vi "Accumulated Correlation 2D.vi"(4 "Microphone Coordinates (cm, rad)":cluster{"r":dbl, "theta":dbl}[](array[cluster]), 5 "Ny":i32=16, 6 "Radius (cm)":dbl=123.4 format="%#_13g", 7 "Nx":i32=16, 8 "Sound Velocity (cm/s)":dbl=576000.0, 9 "Sampling Rate":i32=500000, 11 "Waveforms":waveform(dbl)[](array[waveform])) -> (2 "Source Coordinates (cm, cm)":cluster{"x":dbl, "y":dbl})   [LabVIEW 2013]
uses:
  <vilib>/Waveform/WDTOps.llb/WDT Index Channel DBL.vi
  <vilib>/Analysis/2dsp.llb/1D Cross Correlation (DBL).vi
  <vilib>/Analysis/NI_AALPro.lvlib
panel:
  out "Rxy 2":dbl[][][](array[numeric])
  out "subarray 2":dbl[](array[numeric])
  out "size(s) 2":i32
  out "Rxy":dbl[](array[numeric])
  out "y Coordinates":dbl[](array[numeric])
  out "x Coordinates":dbl[](array[numeric])
  out "Cross Corr.\n1/2 Length":i32
  out "dy":dbl
  out "dx":dbl
  out "Signals":waveform(dbl)[](graph)
  out "subarray":dbl[][](array[numeric])
  out "size(s)":i32[](array[numeric])
  out "Correlation":dbl[][](graph)
  out "Lag Matrix":dbl[][](array[numeric])
  # "Inputs and Outputs"
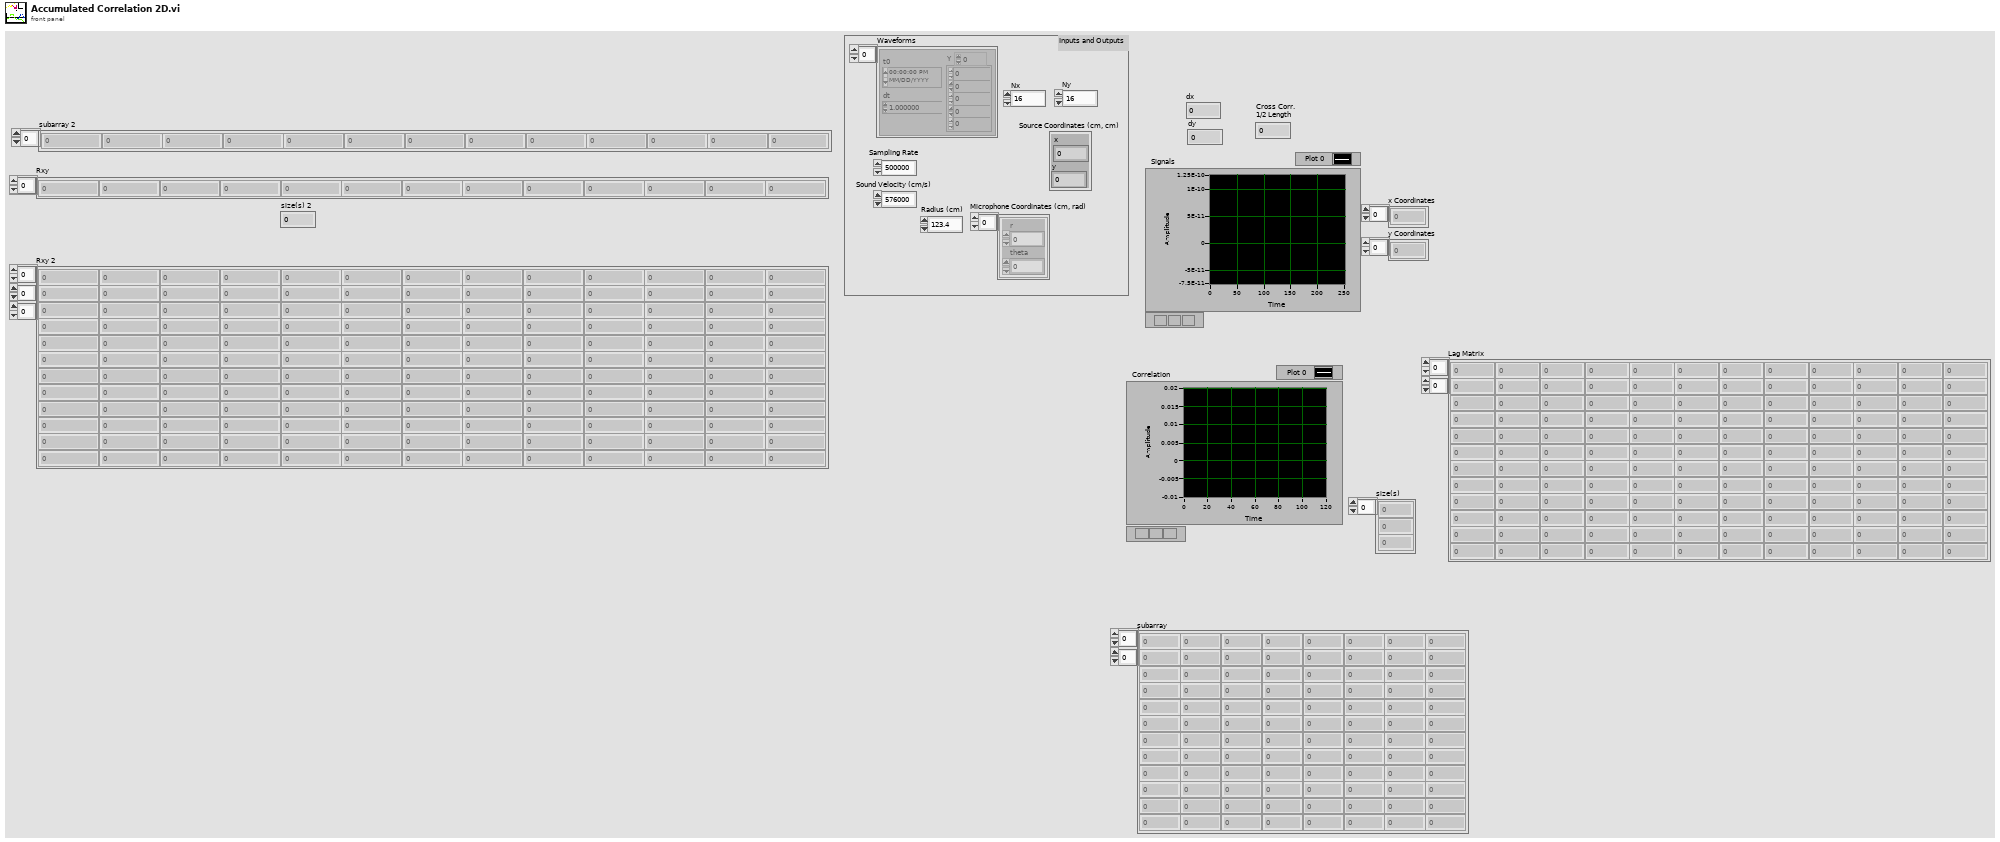
[diagram p1: front panel]
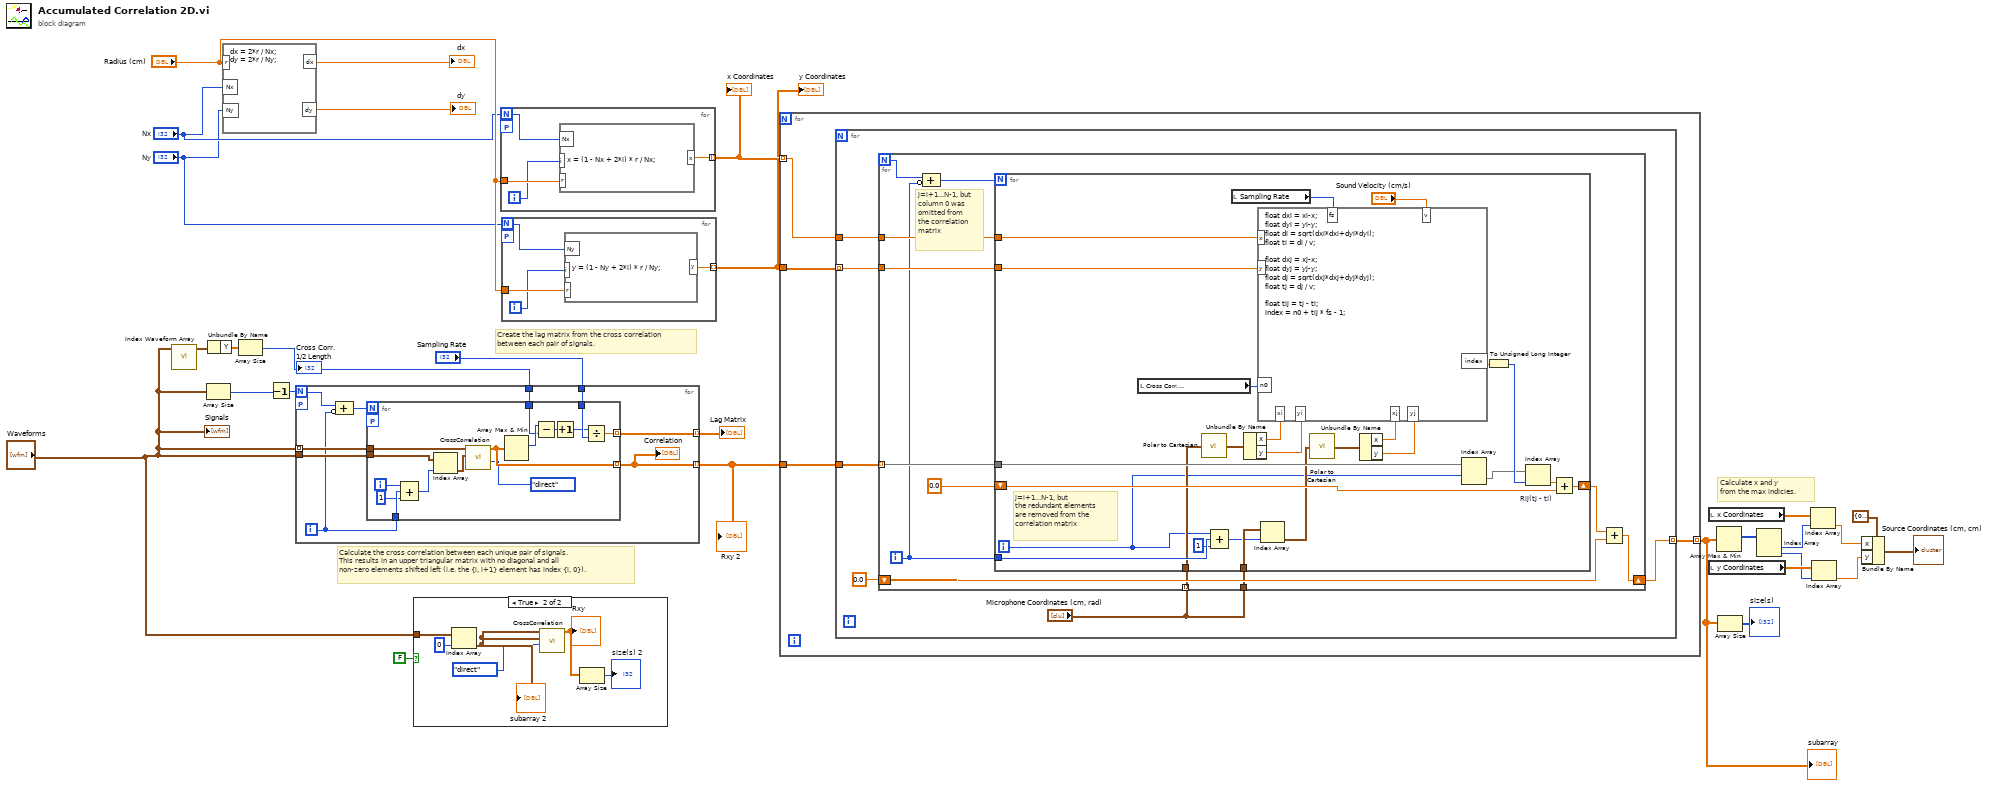
[diagram p0: block diagram]
diagram:
  # "Calculate the cross correlation between each unique pair of signals.\nThis results in an upper triangular matrix with no diagonal and all\nnon-zero elements shifted left (i.e. the {i, i+1} element has index {i, 0})."
  # "Create the lag matrix from the cross correlation\nbetween each pair of signals."
  # "Calculate x and y\nfrom the max indicies."
  n1 = call-poly <vilib>:"Index Waveform Array.vi"("waveform array"="Waveforms") -> ("waveform"=w3:waveform(dbl))  [unwired: 9 in, 1 out]
  n2 = Array Size ("Size(s)")(array="Waveforms") -> (size(s)=w5:i32)
  n3 = Unbundle By Name(w3) -> ("Y"=w2:dbl[])
  n4 = formula code="dx = 2*r / Nx;\ndy = 2*r / Ny;"("r"="Radius (cm)", "Nx"="Nx", "Ny"="Ny") -> ("dx"=→"dx":dbl, "dy"=→"dy":dbl)
  n5 = Array Size(array=w2) -> (size(s)=w1:i32)
  "Cross Corr.\n1/2 Length" <- w1
  n6 = Decrement(x=w5) -> (x-1=w9:i32)
  n7 = for {
    N: w9 -> [w30]
    tunnel: "Waveforms" -> [w33] mode=indexing
    tunnel: "Waveforms" -> [w37]
    tunnel: "Sampling Rate" -> [w36]
    tunnel: [w35] -> w28 mode=indexing
    tunnel: [w34] -> w10 mode=indexing
    tunnel: w1 -> [w32]
    workers-P: _ -> [_]
    i -> [w29]
    n8 = Compound Arithmetic op=ADD(w30, invert w29) -> (w31:i32)
    n9 = for {
      N: w31 -> [_]
      tunnel: w37 -> [w40]
      tunnel: w33 -> [w52]
      tunnel: w36 -> [w51]
      tunnel: [w50] -> w35 mode=indexing
      tunnel: [w47] -> w34 mode=indexing
      tunnel: w32 -> [w45]
      tunnel: w29 -> [w42]
      workers-P: _ -> [_]
      i -> [w43]
      n10 = Compound Arithmetic op=ADD(w43, w42, 1 ("value")) -> (w41:i32)
      n11 = Index Array(array=w40, index=w41) -> (element=w39:waveform(dbl))
      n12 = call-poly <vilib>:"CrossCorrelation.vi"("algorithm"=enum32{"direct", "frequency domain"}."direct", "Y"=w39, "X"=w52) -> ("Rxy"=w47:dbl[])  [unwired: 7 in, 1 out]
      n13 = Array Max & Min(array=w47) -> (max index (indices)=w46:i32)  [unwired: 3 out]
      n14 = Subtract(x=w46, y=w45) -> (x-y=w49:i32)
      n15 = Increment(x=w49) -> (x+1=w48:i32)
      n16 = Divide(x=w48, y=w51) -> (x/y=w50:dbl)
    }
    "Correlation" <- w34
  }
  "Lag Matrix" <- w28
  "Rxy 2" <- w10
  n17 = case shown="True" FALSE {
    tunnel: "Waveforms" -> [_ w58]
    frame False {
    }
    frame True {
      n18 = Index Array(array=w58, index=0 ("index (row)")) -> (element=w56:waveform(dbl))
      "subarray 2" <- w56
      n19 = call-poly <vilib>:"CrossCorrelation.vi"("algorithm"=enum32{"direct", "frequency domain"}."direct", "Y"=w56, "X"=w56) -> ("Rxy"=w54:dbl[])  [unwired: 7 in, 1 out]
      "Rxy" <- w54
      n20 = Array Size(array=w54) -> (size(s)=→"size(s) 2":i32)
    }
  }
  n21 = for {
    N: "Nx" -> [w59]
    tunnel: "Radius (cm)" -> [w62]
    tunnel: [w60] -> w18 mode=indexing
    workers-P: _ -> [_]
    i -> [w61]
    n22 = formula code="x = (1 - Nx + 2*i) * r / Nx;"("r"=w62, "i"=w61, "Nx"=w59) -> ("x"=w60:dbl)
  }
  "x Coordinates" <- w18
  n23 = for {
    N: "Ny" -> [w63]
    tunnel: "Radius (cm)" -> [w66]
    tunnel: [w64] -> w17 mode=indexing
    workers-P: _ -> [_]
    i -> [w65]
    n24 = formula code="y = (1 - Ny + 2*i) * r / Ny;"("r"=w66, "i"=w65, "Ny"=w63) -> ("y"=w64:dbl)
  }
  "y Coordinates" <- w17
  n25 = for {
    tunnel: [w70] -> w25 mode=indexing
    tunnel: w10 -> [w69]
    tunnel: w18 -> [w67] mode=indexing
    tunnel: w17 -> [w68]
    n26 = for {
      tunnel: [w75] -> w70 mode=indexing
      tunnel: w69 -> [w74]
      tunnel: w68 -> [w72] mode=indexing
      tunnel: w67 -> [w71]
      n27 = for {
        N -> [w81]
        shift-right: [w86] -> w75
        shift-left: 0.0 -> [w87]
        tunnel: "Microphone Coordinates (cm, rad)" -> [w85] mode=indexing
        tunnel: "Microphone Coordinates (cm, rad)" -> [w80]
        tunnel: w74 -> [w78] mode=indexing
        tunnel: w71 -> [w83]
        tunnel: w72 -> [w82]
        i -> [w77]
        # "j=i+1...N-1, but\ncolumn 0 was\nomitted from\nthe correlation\nmatrix"
        n28 = Compound Arithmetic op=ADD(w81, invert w77) -> (w79:i32)
        n29 = for {
          N: w79 -> [_]
          shift-right: [w111] -> w88
          shift-left: 0.0 -> [w109]
          tunnel: w80 -> [w95]
          tunnel: w85 -> [w92]
          tunnel: w78 -> [w96]
          tunnel: w83 -> [w99]
          tunnel: w82 -> [w98]
          tunnel: w77 -> [w97]
          i -> [w89]
          # "j=i+1...N-1, but\nthe redundant elements\nare removed from the\ncorrelation matrix"
          n30 = local read "Cross Corr.\n1/2 Length"() -> (w100:i32)
          n31 = call "Polar to Cartesian.vi"("Polar\nCoordinates"=w92) -> ("Cartesian\nCoordinates"=w106:cluster{"x":dbl, "y":dbl})  [unwired: 4 in]
          n32 = Compound Arithmetic op=ADD(w89, w97, 1 ("value")) -> (w91:i32)
          n33 = local read "Sampling Rate"() -> (w108:i32)
          n34 = Unbundle By Name(w106) -> ("x"=w105:dbl, "y"=w104:dbl)
          n35 = Index Array(array=w95, index=w91) -> (element=w94:cluster{"r":dbl, "theta":dbl})
          n36 = call "Polar to Cartesian.vi"("Polar\nCoordinates"=w94) -> ("Cartesian\nCoordinates"=w103:cluster{"x":dbl, "y":dbl})  [unwired: 4 in]
          n37 = Unbundle By Name(w103) -> ("x"=w102:dbl, "y"=w101:dbl)
          n38 = formula code="float dxi = xi-x;\nfloat dyi = yi-y;\nfloat di = sqrt(dxi*dxi+dyi*dyi);\nfloat ti = di / v;\n\nfloat dxj = xj-x;\nfloat dyj = yj-y;\nfloat dj = sqrt(dxj*dxj+dyj*dyj);\nfloat tj = dj / v;\n\nfloat tij = tj - ti;\nindex = n0 + tij * fs - 1;"("xi"=w105, "yi"=w104, "xj"=w102, "yj"=w101, "x"=w99, "y"=w98, "v"="Sound Velocity (cm/s)", "fs"=w108, "n0"=w100) -> ("index"=w113:dbl)
          n39 = Index Array(array=w96, index (row)=w89) -> (element=w93:dbl[])  [unwired: 1 in]
          n40 = To Unsigned Long Integer(number=w113) -> (unsigned 32bit integer=w112:u32)
          n41 = Index Array "Rij(tj - ti)"(array=w93, index=w112) -> (element=w110:dbl)
          n42 = Add(x=w110, y=w109) -> (x+y=w111:dbl)
        }
        n43 = Add(x=w88, y=w87) -> (x+y=w86:dbl)
      }
    }
  }
  "subarray" <- w25
  n44 = local read "x Coordinates"() -> (w16:dbl[])
  n45 = local read "y Coordinates"() -> (w14:dbl[])
  n46 = Array Max & Min(array=w25) -> (max index (indices)=w27:i32[])  [unwired: 3 out]
  n47 = Array Size(array=w25) -> (size(s)=→"size(s)":i32[])
  n48 = Index Array(array=w27) -> (element #1=w15:i32, element #2=w13:i32)  [unwired: 2 in]
  n49 = Index Array(array=w16, index=w15) -> (element=w11:dbl)
  n50 = Index Array(array=w14, index=w13) -> (element=w12:dbl)
  n51 = Bundle By Name(cluster=cluster{"x":dbl, "y":dbl} {"x"=0.0, "y"=0.0} ("Polar\nCoordinates"), "x"=w11, "y"=w12) -> (→"Source Coordinates (cm, cm)":cluster{"x":dbl, "y":dbl})
  "Signals" <- "Waveforms"
